vi "Calc_Tipper.vi"(11 "Tipper Command Inputs":T1) -> (3 "Bridge Tipper Outputs":T2)   [LabVIEW 2012]
uses:
  Outputs_Tipper.ctl
  Inputs_Tipper.ctl
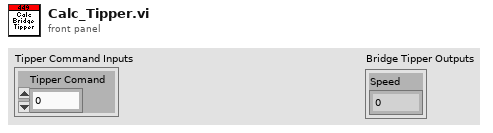
[diagram p1: front panel]
types:
  T1 = typedef "Inputs_Tipper.ctl" = cluster{"Tipper Comand":dbl}
  T2 = typedef "Outputs_Tipper.ctl" = cluster{"Speed":dbl}
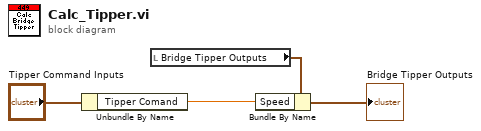
[diagram p0: block diagram]
diagram:
  n1 = Unbundle By Name("Tipper Command Inputs") -> ("Tipper Comand"=w1:dbl)
  n2 = local read "Bridge Tipper Outputs"() -> (w4:T2)
  n3 = Bundle By Name(cluster=w4, "Speed"=w1) -> (→"Bridge Tipper Outputs":T2)
